vi "CRYRead Weighting.vi"(10 "Weighting filename":string) -> (3 "Array":cluster{dbl, dbl, dbl}[](array[cluster]))   [LabVIEW 2013]
uses:
  CRYMainGlobal.vi
panel:
  out "Weight [Hz,dB]":cluster{dbl, dbl}[](array[cluster])=[{100.0, 154.0}, {125.0, 115.4}, {160.0, 89.0}, {200.0, 77.2}, {315.0, 62.3}, {400.0, 45.0}, {500.0, 53.4}, {630.0, 48.8}, {800.0, 47.9}, {1000.0, 50.4}, {1250.0, 59.4}, {1600.0, 57.0}, {2000.0, 72.5}, {2500.0, 72.9}, {3150.0, 89.5}, {4000.0, 117.3}, {5000.0, 157.3}, {6300.0, 172.2}, {8000.0, 181.7}] {"?" format="%.2f"; "?" format="%.2f"}
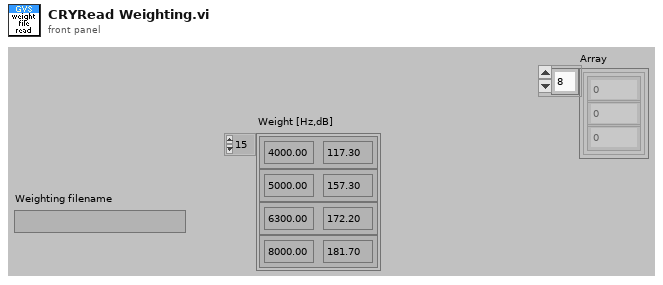
[diagram p1: front panel]
types:
  T1 = enum16{"read/write", "read-only", "write-only", "write-only (truncate)"}
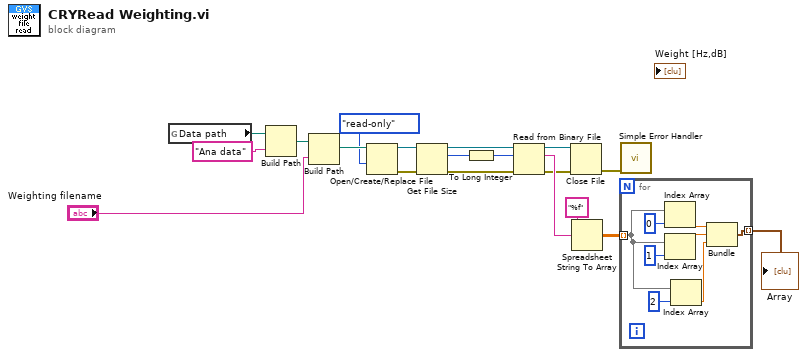
[diagram p0: block diagram]
diagram:
  n1 = global read "CRYMainGlobal.vi" "Data path"() -> (w2:path)
  n2 = Build Path(base path=w2, name or relative path="Ana data") -> (appended path=w3:path)
  n3 = Build Path(base path=w3, name or relative path="Weighting filename") -> (appended path=w18:path)
  n4 = Open/Create/Replace File(file path (use dialog)=w18, access (0:read/write)=T1."read-only" ("open mode (0)")) -> (refnum out=w15:refnum<file>, error out=w16:errorcluster)  [unwired: 1 in, 4 out]
  n5 = Get File Size(file=w15, error in=w16) -> (refnum out=w12:refnum<file>, size (in bytes)=w5:i64, 0:w13:errorcluster)
  n6 = To Long Integer(number=w5) -> (32bit integer=w14:i32)
  n7 = Read from Binary File(8:w13, 10:w14, 11:w12) -> (0:w10:errorcluster, 2:w11:string, 3:w9:refnum<file>)  [unwired: 4 out]
  n8 = Close File(refnum=w9, error in=w10) -> (error out=w6:errorcluster)  [unwired: 1 out]
  n9 = Spreadsheet String To Array(format string="%f", spreadsheet string=w11) -> (array=w7:dbl[][])  [unwired: 2 out]
  n10 = for {
    tunnel: w7 -> [w21] mode=indexing
    tunnel: [w23] -> w1 mode=indexing
    n11 = Index Array(array=w21, index=0 ("Index")) -> (element=w25:dbl)
    n12 = Index Array(array=w21, index=1 ("Index")) -> (element=w24:dbl)
    n13 = Index Array(array=w21, index=2 ("Index")) -> (element=w20:dbl)
    n14 = Bundle(w25, w24, w20) -> (w23:cluster{dbl, dbl, dbl})  [unwired: 1 out]
  }
  "Array" <- w1
  n15 = call <vilib>:"Simple Error Handler.vi"("error in (no error)"=w6) -> ()  [unwired: 1 in, 8 out]
